vi "getAnonymousCredentials.vi"(11 "Connection.NetworkStream":refnum<class "Connection.NetworkStream.lvclass">) -> (1 "Anonymous password":string, 2 "Anonymous username":string)   [LabVIEW 2013, in "Connection.NetworkQueue_GOSPL.lvlib" / "Connection.NetworkStream.lvclass"]
uses:
  Connection.NetworkStream/Connection.NetworkStream.lvclass
  Store/Store.lvclass
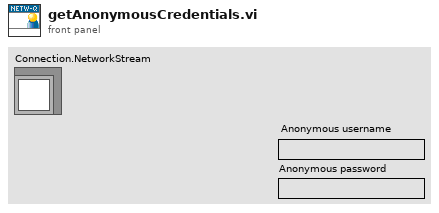
[diagram p1: front panel]
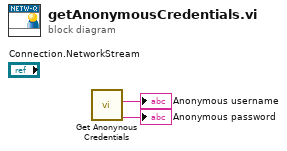
[diagram p0: block diagram]
diagram:
  n1 = call "Get Anonynous Credentials.vi"() -> ("Anonymous password"=→"Anonymous password":string, "Anonymous username"=→"Anonymous username":string)  [unwired: 10 in]
